vi "InitializeMotorsXYZR_V2.vi"(0 "COM PORT Array IN":refnum<visa-resource-name>[](array[refnum]), 1 "STEP SP Array IN":i32[](array[numeric]), 2 "XYZ in RANGE Array IN":bool[](array[boolean]), 3 "XYZR VEL PV Array IN":i32[](array[numeric]), 4 "RUNHOLDArray IN":i32[](array[numeric]), 5 "Error Array IN":errorcluster[](array[cluster]), 6 "ZR Max Min array":dbl[](array[numeric])) -> (13 "XY Max Min array OUT":dbl[](array[numeric]), 14 "COM PORT Array OUT":refnum<visa-resource-name>[](array[refnum]), 15 "STEP SP Array OUT":i32[](array[numeric]), 16 "XYZ in RANGE Array OUT":bool[](array[boolean]), 17 "XYZR VEL PV Array OUT":i32[](array[numeric]), 18 "XYZR MAX MIN POS":i32[](array[numeric]), 19 "Error Array OUT":errorcluster[](array[cluster]))   [LabVIEW 2010]
panel:
  out "R velocity PV step/sec[3]":i32
  out "Z velocity PV step/sec[2]":i32
  out "Y velocity PV step/sec[1]":i32
  out "X velocity PV step/sec[0]":i32
  out "R in Range[3]":bool
  out "Z in Range[2]":bool
  out "Y in Range[1]":bool
  out "X in Range[0]":bool
  out "R Step SP[3]":i32
  out "Z Step SP[2]":i32
  out "Y Step SP[1]":i32 min=-2304000 max=2304000
  out "X Velocity SP step/sec[4]":i32
  out "Y Velocity SP step/sec[5]":i32
  out "Z Velocity SP step/sec[6]":i32
  out "R Velocity SP step/sec[7]":i32
  out "X Step SP[0]":i32 min=-2304000 max=2304000
  out "Z Run Holding %[7]":i32
  out "R Run Current %[6]":i32
  out "R Run Holding %[5]":i32
  out "Y Run Current %[4]":i32
  out "Y Run Holding %[3]":i32
  out "Z Run Current %[2]":i32
  out "X Run Holding %[1]":i32
  out "X Run Current %[0]":i32
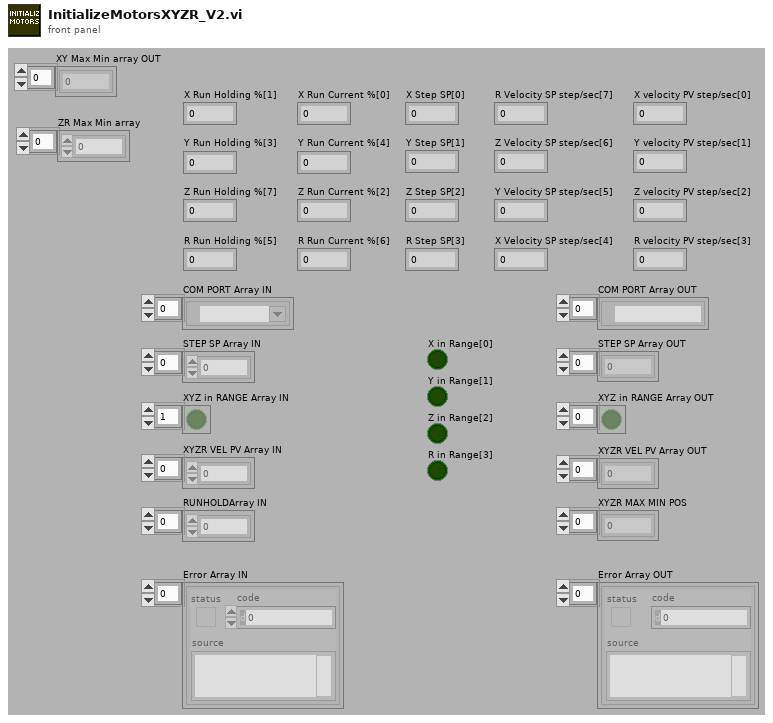
[diagram p1: front panel]
types:
  T1 = cluster{"XYZR VEL PV Array IN[0]":i32, "XYZR VEL PV Array IN[1]":i32, "XYZR VEL PV Array IN[2]":i32, "XYZR VEL PV Array IN[3]":i32, "XYZR VEL PV Array IN[4]":i32, "XYZR VEL PV Array IN[5]":i32, "XYZR VEL PV Array IN[6]":i32, "XYZR VEL PV Array IN[7]":i32, "XYZR VEL PV Array IN[8]":i32}
  T2 = cluster{"RUNHOLDArray IN[0]":i32, "RUNHOLDArray IN[1]":i32, "RUNHOLDArray IN[2]":i32, "RUNHOLDArray IN[3]":i32, "RUNHOLDArray IN[4]":i32, "RUNHOLDArray IN[5]":i32, "RUNHOLDArray IN[6]":i32, "RUNHOLDArray IN[7]":i32, "RUNHOLDArray IN[8]":i32}
  T3 = cluster{"STEP SP Array IN[0]":i32, "STEP SP Array IN[1]":i32, "STEP SP Array IN[2]":i32, "STEP SP Array IN[3]":i32, "STEP SP Array IN[4]":i32, "STEP SP Array IN[5]":i32, "STEP SP Array IN[6]":i32, "STEP SP Array IN[7]":i32, "STEP SP Array IN[8]":i32}
  T4 = cluster{"XYZ in RANGE Array IN[0]":bool, "XYZ in RANGE Array IN[1]":bool, "XYZ in RANGE Array IN[2]":bool, "XYZ in RANGE Array IN[3]":bool, "XYZ in RANGE Array IN[4]":bool, "XYZ in RANGE Array IN[5]":bool, "XYZ in RANGE Array IN[6]":bool, "XYZ in RANGE Array IN[7]":bool, "XYZ in RANGE Array IN[8]":bool}
  T5 = cluster{"RUNHOLDArray IN[0]":i32, "RUNHOLDArray IN[4]":i32}
  T6 = cluster{"RUNHOLDArray IN[2]":i32, "RUNHOLDArray IN[6]":i32}
  T7 = cluster{"RUNHOLDArray IN[1]":i32, "RUNHOLDArray IN[3]":i32}
  T8 = cluster{"RUNHOLDArray IN[7]":i32, "RUNHOLDArray IN[5]":i32}
  T9 = cluster{"STEP SP Array IN[4]":i32, "STEP SP Array IN[5]":i32}
  T10 = cluster{"STEP SP Array IN[6]":i32, "STEP SP Array IN[7]":i32}
  T11 = cluster{"COM PORT Array IN[0]":refnum<visa-resource-name>, "COM PORT Array IN[1]":refnum<visa-resource-name>, "COM PORT Array IN[2]":refnum<visa-resource-name>, "COM PORT Array IN[3]":refnum<visa-resource-name>, "COM PORT Array IN[4]":refnum<visa-resource-name>, "COM PORT Array IN[5]":refnum<visa-resource-name>, "COM PORT Array IN[6]":refnum<visa-resource-name>, "COM PORT Array IN[7]":refnum<visa-resource-name>, "COM PORT Array IN[8]":refnum<visa-resource-name>}
  T12 = cluster{"Error Array IN[0]":errorcluster, "Error Array IN[1]":errorcluster, "Error Array IN[2]":errorcluster, "Error Array IN[3]":errorcluster, "Error Array IN[4]":errorcluster, "Error Array IN[5]":errorcluster, "Error Array IN[6]":errorcluster, "Error Array IN[7]":errorcluster, "Error Array IN[8]":errorcluster}
  T13 = cluster{"ZR Max Min array[0]":dbl, "ZR Max Min array[1]":dbl, "ZR Max Min array[2]":dbl, "ZR Max Min array[3]":dbl, "ZR Max Min array[4]":dbl, "ZR Max Min array[5]":dbl, "ZR Max Min array[6]":dbl, "ZR Max Min array[7]":dbl, "ZR Max Min array[8]":dbl}
  T14 = cluster{"ZR Max Min array[0]":dbl, "ZR Max Min array[2]":dbl}
  T15 = cluster{"ZR Max Min array[1]":dbl, "ZR Max Min array[3]":dbl}
  T16 = cluster{"COM PORT Array IN[0]":refnum<visa-resource-name>, "COM PORT Array IN[2]":refnum<visa-resource-name>}
  T17 = cluster{"Error Array IN[0]":errorcluster, "Error Array IN[2]":errorcluster}
  T18 = cluster{"COM PORT Array IN[1]":refnum<visa-resource-name>, "COM PORT Array IN[3]":refnum<visa-resource-name>}
  T19 = cluster{"Error Array IN[1]":errorcluster, "Error Array IN[3]":errorcluster}
  T20 = enum16{"Stop", "Reset", "Run Current", "Holding Current", "Accel Rate", "Decel Rate", "Move to Relative Position", "Move to Absolute Position", "Echo Mode", "Print Parameter", "Send String", "Microstep Resolution", "Set Current Position", "Max Velocity"}
  T21 = cluster{"[0]":i32, "[1]":i32, "[2]":i32, "[3]":i32, "[4]":i32, "[5]":i32, "[6]":i32, "[7]":i32, "[8]":i32}
  T22 = cluster{"[0]":refnum<visa-resource-name>, "[1]":refnum<visa-resource-name>, "[2]":refnum<visa-resource-name>, "[3]":refnum<visa-resource-name>, "[4]":refnum<visa-resource-name>, "[5]":refnum<visa-resource-name>, "[6]":refnum<visa-resource-name>, "[7]":refnum<visa-resource-name>, "[8]":refnum<visa-resource-name>}
  T23 = cluster{"[0]":errorcluster, "[1]":errorcluster, "[2]":errorcluster, "[3]":errorcluster, "[4]":errorcluster, "[5]":errorcluster, "[6]":errorcluster, "[7]":errorcluster, "[8]":errorcluster}
  T24 = cluster{"[0]":dbl, "[1]":dbl, "[2]":dbl, "[3]":dbl, "[4]":dbl, "[5]":dbl, "[6]":dbl, "[7]":dbl, "[8]":dbl}
  T25 = cluster{"[0]":bool, "[1]":bool, "[2]":bool, "[3]":bool, "[4]":bool, "[5]":bool, "[6]":bool, "[7]":bool, "[8]":bool}
  T26 = cluster{"[0]":dbl, "[0]":dbl, "[1]":dbl, "[1]":dbl}
  T27 = cluster{"[0]":bool, "[1]":bool, "[0]":bool, "[1]":bool}
  T28 = cluster{"[0]":i32, "[0]":i32, "[1]":i32, "[1]":i32, "[0]":i32, "[0]":i32, "[1]":i32, "[1]":i32}
  T29 = cluster{"[0]":i32, "[1]":i32, "[0]":i32, "[1]":i32}
  T30 = cluster{"[0]":refnum<visa-resource-name>, "[0]":refnum<visa-resource-name>, "[1]":refnum<visa-resource-name>, "[1]":refnum<visa-resource-name>}
  T31 = cluster{"[0]":errorcluster, "[0]":errorcluster, "[1]":errorcluster, "[1]":errorcluster}
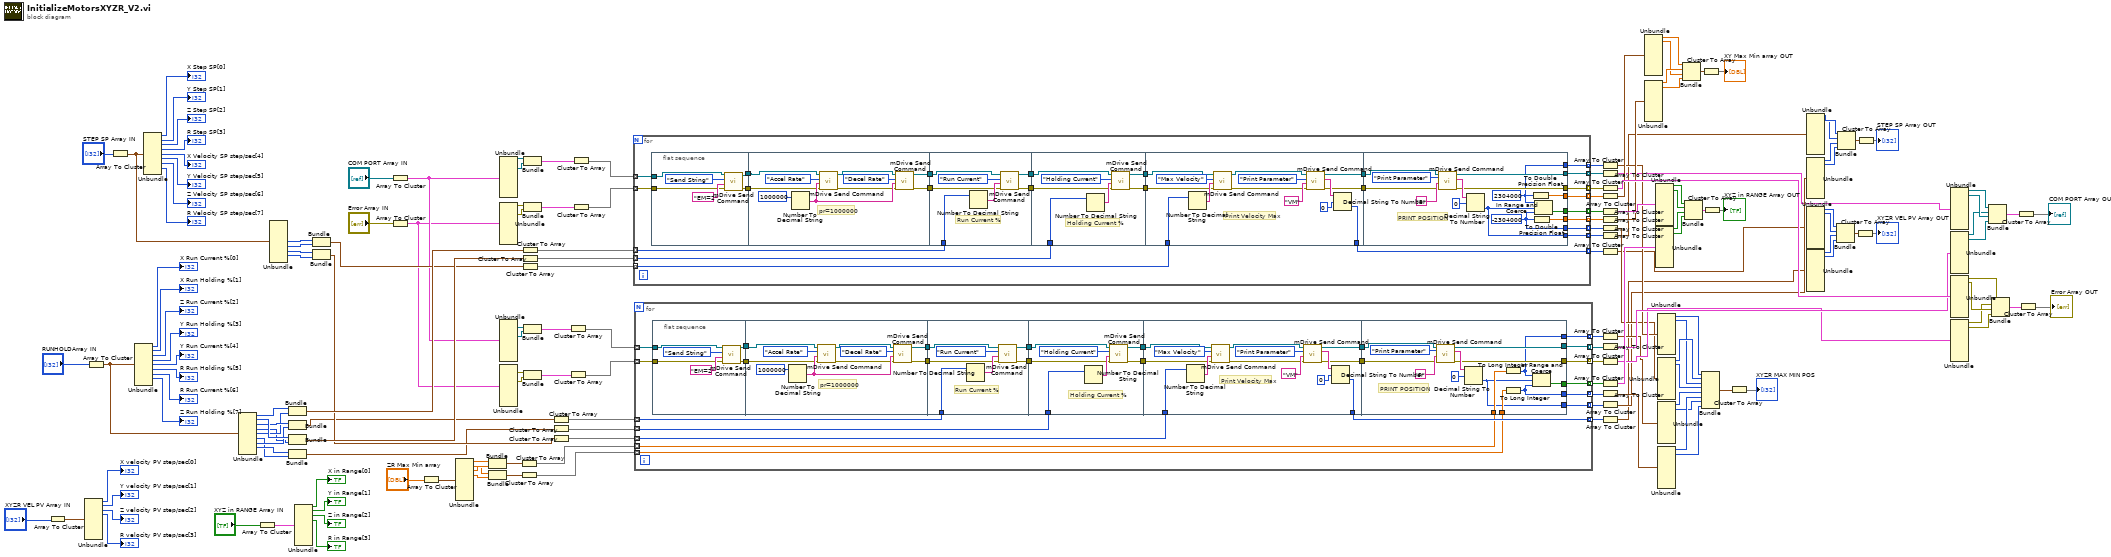
[diagram p0: block diagram]
diagram:
  n1 = Array To Cluster(array="XYZR VEL PV Array IN") -> (cluster=w148:T1)
  n2 = Unbundle(w148) -> ("XYZR VEL PV Array IN[0]"=→"X velocity PV step/sec[0]":i32, "XYZR VEL PV Array IN[1]"=→"Y velocity PV step/sec[1]":i32, "XYZR VEL PV Array IN[2]"=→"Z velocity PV step/sec[2]":i32, "XYZR VEL PV Array IN[3]"=→"R velocity PV step/sec[3]":i32)  [unwired: 5 out]
  n3 = Array To Cluster(array="RUNHOLDArray IN") -> (cluster=w120:T2)
  n4 = Array To Cluster(array="STEP SP Array IN") -> (cluster=w115:T3)
  n5 = Unbundle(w120) -> ("RUNHOLDArray IN[0]"=→"X Run Current %[0]":i32, "RUNHOLDArray IN[1]"=→"X Run Holding %[1]":i32, "RUNHOLDArray IN[2]"=→"Z Run Current %[2]":i32, "RUNHOLDArray IN[3]"=→"Y Run Holding %[3]":i32, "RUNHOLDArray IN[4]"=→"Y Run Current %[4]":i32, "RUNHOLDArray IN[5]"=→"R Run Holding %[5]":i32, "RUNHOLDArray IN[6]"=→"R Run Current %[6]":i32, "RUNHOLDArray IN[7]"=→"Z Run Holding %[7]":i32)  [unwired: 1 out]
  n6 = Unbundle(w115) -> ("STEP SP Array IN[0]"=→"X Step SP[0]":i32, "STEP SP Array IN[1]"=→"Y Step SP[1]":i32, "STEP SP Array IN[2]"=→"Z Step SP[2]":i32, "STEP SP Array IN[3]"=→"R Step SP[3]":i32, "STEP SP Array IN[4]"=→"X Velocity SP step/sec[4]":i32, "STEP SP Array IN[5]"=→"Y Velocity SP step/sec[5]":i32, "STEP SP Array IN[6]"=→"Z Velocity SP step/sec[6]":i32, "STEP SP Array IN[7]"=→"R Velocity SP step/sec[7]":i32)  [unwired: 1 out]
  n7 = Unbundle(w120) -> ("RUNHOLDArray IN[0]"=w113:i32, "RUNHOLDArray IN[1]"=w112:i32, "RUNHOLDArray IN[2]"=w92:i32, "RUNHOLDArray IN[3]"=w89:i32, "RUNHOLDArray IN[4]"=w91:i32, "RUNHOLDArray IN[5]"=w87:i32, "RUNHOLDArray IN[6]"=w90:i32, "RUNHOLDArray IN[7]"=w88:i32)  [unwired: 1 out]
  n8 = Array To Cluster(array="XYZ in RANGE Array IN") -> (cluster=w149:T4)
  n9 = Unbundle(w115) -> ("STEP SP Array IN[4]"=w114:i32, "STEP SP Array IN[5]"=w96:i32, "STEP SP Array IN[6]"=w95:i32, "STEP SP Array IN[7]"=w94:i32)  [unwired: 5 out]
  n10 = Bundle("RUNHOLDArray IN[0]"=w113, "RUNHOLDArray IN[4]"=w91) -> (w119:T5)  [unwired: 1 in]
  n11 = Bundle("RUNHOLDArray IN[2]"=w92, "RUNHOLDArray IN[6]"=w90) -> (w85:T6)  [unwired: 1 in]
  n12 = Bundle("RUNHOLDArray IN[1]"=w112, "RUNHOLDArray IN[3]"=w89) -> (w118:T7)  [unwired: 1 in]
  n13 = Bundle("RUNHOLDArray IN[7]"=w88, "RUNHOLDArray IN[5]"=w87) -> (w84:T8)  [unwired: 1 in]
  n14 = Unbundle(w149) -> ("XYZ in RANGE Array IN[0]"=→"X in Range[0]":bool, "XYZ in RANGE Array IN[1]"=→"Y in Range[1]":bool, "XYZ in RANGE Array IN[2]"=→"Z in Range[2]":bool, "XYZ in RANGE Array IN[3]"=→"R in Range[3]":bool)  [unwired: 5 out]
  n15 = Bundle("STEP SP Array IN[4]"=w114, "STEP SP Array IN[5]"=w96) -> (w111:T9)  [unwired: 1 in]
  n16 = Bundle("STEP SP Array IN[6]"=w95, "STEP SP Array IN[7]"=w94) -> (w93:T10)  [unwired: 1 in]
  n17 = Array To Cluster(array="COM PORT Array IN") -> (cluster=w109:T11)
  n18 = Array To Cluster(array="Error Array IN") -> (cluster=w108:T12)
  n19 = Array To Cluster(array="ZR Max Min array") -> (cluster=w75:T13)
  n20 = Unbundle(w75) -> ("ZR Max Min array[0]"=w74:dbl, "ZR Max Min array[1]"=w72:dbl, "ZR Max Min array[2]"=w73:dbl, "ZR Max Min array[3]"=w71:dbl)  [unwired: 5 out]
  n21 = Bundle("ZR Max Min array[0]"=w74, "ZR Max Min array[2]"=w73) -> (w70:T14)  [unwired: 1 in]
  n22 = Bundle("ZR Max Min array[1]"=w72, "ZR Max Min array[3]"=w71) -> (w69:T15)  [unwired: 1 in]
  n23 = Unbundle(w109) -> ("COM PORT Array IN[0]"=w107:refnum<visa-resource-name>, "COM PORT Array IN[2]"=w80:refnum<visa-resource-name>)  [unwired: 7 out]
  n24 = Unbundle(w108) -> ("Error Array IN[0]"=w106:errorcluster, "Error Array IN[2]"=w79:errorcluster)  [unwired: 7 out]
  n25 = Unbundle(w109) -> ("COM PORT Array IN[1]"=w78:refnum<visa-resource-name>, "COM PORT Array IN[3]"=w105:refnum<visa-resource-name>)  [unwired: 7 out]
  n26 = Unbundle(w108) -> ("Error Array IN[1]"=w77:errorcluster, "Error Array IN[3]"=w81:errorcluster)  [unwired: 7 out]
  n27 = Cluster To Array(cluster=w70) -> (array=w68:dbl[])
  n28 = Cluster To Array(cluster=w69) -> (array=w67:dbl[])
  n29 = Cluster To Array(cluster=w119) -> (array=w117:i32[])
  n30 = Cluster To Array(cluster=w118) -> (array=w116:i32[])
  n31 = Cluster To Array(cluster=w111) -> (array=w110:i32[])
  n32 = Bundle("COM PORT Array IN[0]"=w107, "COM PORT Array IN[2]"=w80) -> (w104:T16)  [unwired: 1 in]
  n33 = Bundle("Error Array IN[0]"=w106, "Error Array IN[2]"=w79) -> (w102:T17)  [unwired: 1 in]
  n34 = Bundle("COM PORT Array IN[1]"=w78, "COM PORT Array IN[3]"=w105) -> (w100:T18)  [unwired: 1 in]
  n35 = Bundle("Error Array IN[1]"=w77, "Error Array IN[3]"=w81) -> (w99:T19)  [unwired: 1 in]
  n36 = Cluster To Array(cluster=w85) -> (array=w82:i32[])
  n37 = Cluster To Array(cluster=w84) -> (array=w83:i32[])
  n38 = Cluster To Array(cluster=w93) -> (array=w86:i32[])
  n39 = Cluster To Array(cluster=w100) -> (array=w97:refnum<visa-resource-name>[])
  n40 = Cluster To Array(cluster=w99) -> (array=w98:errorcluster[])
  n41 = Cluster To Array(cluster=w104) -> (array=w103:refnum<visa-resource-name>[])
  n42 = Cluster To Array(cluster=w102) -> (array=w101:errorcluster[])
  n43 = for {
    tunnel: w103 -> [w186] mode=indexing
    tunnel: w101 -> [w185] mode=indexing
    tunnel: w117 -> [w182] mode=indexing
    tunnel: w116 -> [w179] mode=indexing
    tunnel: w110 -> [w176] mode=indexing
    tunnel: [w173] -> w65 mode=indexing
    tunnel: [w172] -> w63 mode=indexing
    tunnel: [w171] -> w62 mode=indexing
    tunnel: [w170] -> w66 mode=indexing
    tunnel: [w169] -> w61 mode=indexing
    tunnel: [w168] -> w60 mode=indexing
    tunnel: [w167] -> w59 mode=indexing
    tunnel: [w166] -> w58 mode=indexing
    tunnel: [w165] -> w64 mode=indexing
    n44 = flat-sequence {
      tunnel: [w192] -> w188
      tunnel: [w191] -> w187
      tunnel: w186 -> [w190]
      tunnel: w185 -> [w189]
      tunnel: w188 -> [w197]
      tunnel: w187 -> [w198]
      tunnel: [w196] -> w184
      tunnel: [w195] -> w183
      tunnel: w184 -> [w208]
      tunnel: w183 -> [w209]
      tunnel: w182 -> [w207]
      tunnel: [w206] -> w181
      tunnel: [w205] -> w180
      tunnel: w181 -> [w216]
      tunnel: w180 -> [w215]
      tunnel: w179 -> [w214]
      tunnel: [w213] -> w178
      tunnel: [w212] -> w177
      tunnel: w178 -> [w223]
      tunnel: w177 -> [w224]
      tunnel: w176 -> [w222]
      tunnel: [w221] -> w175
      tunnel: [w220] -> w174
      tunnel: [w219] -> w173
      tunnel: w175 -> [w242]
      tunnel: w174 -> [w241]
      tunnel: [w240] -> w168
      tunnel: [w239] -> w167
      tunnel: [w238] -> w171
      tunnel: [w237] -> w172
      tunnel: [w236] -> w166
      tunnel: [w235] -> w170
      tunnel: [w234] -> w169
      tunnel: [w233] -> w165
      frame #0 {
        n45 = call "mDrive Send Command.vi"("error in (no error)"=w189, "Extra"="EM=2", "Command"=T20."Send String", "VISA resource name"=w190) -> ("error out"=w192:errorcluster, "VISA resource name out"=w191:refnum<visa-resource-name>)  [unwired: 3 in, 1 out]
      }
      frame #1 {
        # "pr=1000000"
        n46 = Number To Decimal String(number=1000000) -> (decimal integer string=w200:string)  [unwired: 1 in]
        n47 = call "mDrive Send Command.vi"("error in (no error)"=w197, "Extra"=w200, "Command"=T20."Accel Rate", "VISA resource name"=w198) -> ("error out"=w199:errorcluster, "VISA resource name out"=w204:refnum<visa-resource-name>)  [unwired: 3 in, 1 out]
        n48 = call "mDrive Send Command.vi"("error in (no error)"=w199, "Extra"=w200, "Command"=T20."Decel Rate", "VISA resource name"=w204) -> ("error out"=w195:errorcluster, "VISA resource name out"=w196:refnum<visa-resource-name>)  [unwired: 3 in, 1 out]
      }
      frame #2 {
        # "Run Current %"
        n49 = Number To Decimal String(number=w207) -> (decimal integer string=w210:string)  [unwired: 1 in]
        n50 = call "mDrive Send Command.vi"("error in (no error)"=w209, "Extra"=w210, "Command"=T20."Run Current", "VISA resource name"=w208) -> ("error out"=w206:errorcluster, "VISA resource name out"=w205:refnum<visa-resource-name>)  [unwired: 3 in, 1 out]
      }
      frame #3 {
        # "Holding Current %"
        n51 = Number To Decimal String(number=w214) -> (decimal integer string=w217:string)  [unwired: 1 in]
        n52 = call "mDrive Send Command.vi"("error in (no error)"=w216, "Extra"=w217, "Command"=T20."Holding Current", "VISA resource name"=w215) -> ("error out"=w212:errorcluster, "VISA resource name out"=w213:refnum<visa-resource-name>)  [unwired: 3 in, 1 out]
      }
      frame #4 {
        # "Print Velocity Max"
        n53 = Number To Decimal String(number=w222) -> (decimal integer string=w228:string)  [unwired: 1 in]
        n54 = call "mDrive Send Command.vi"("error in (no error)"=w224, "Extra"=w228, "Command"=T20."Max Velocity", "VISA resource name"=w223) -> ("error out"=w229:errorcluster, "VISA resource name out"=w225:refnum<visa-resource-name>)  [unwired: 3 in, 1 out]
        n55 = call "mDrive Send Command.vi"("error in (no error)"=w229, "Extra"="VM", "Command"=T20."Print Parameter", "VISA resource name"=w225) -> ("error out"=w220:errorcluster, "read buffer"=w227:string, "VISA resource name out"=w221:refnum<visa-resource-name>)  [unwired: 3 in]
        n56 = Decimal String To Number(string=w227, offset=0) -> (number=w219:i32)  [unwired: 1 in, 1 out]
      }
      frame #5 {
        w237 = -2304000 ("lower limit")
        w236 = 2304000 ("upper limit")
        # "PRINT POSITION"
        n57 = call "mDrive Send Command.vi"("error in (no error)"=w241, "Extra"="P", "Command"=T20."Print Parameter", "VISA resource name"=w242) -> ("error out"=w240:errorcluster, "read buffer"=w243:string, "VISA resource name out"=w239:refnum<visa-resource-name>)  [unwired: 3 in]
        n58 = Decimal String To Number(string=w243, offset=0) -> (number=w233:i32)  [unwired: 1 in, 1 out]
        n59 = To Double Precision Float(number=w236) -> (double precision float=w234:dbl)
        n60 = To Double Precision Float(number=w237) -> (double precision float=w238:dbl)
        n61 = In Range and Coerce(upper limit=w236, x=w233, lower limit=w237) -> (In Range?=w235:bool)  [unwired: 1 out]
      }
    }
  }
  n62 = for {
    tunnel: [w260] -> w51 mode=indexing
    tunnel: w98 -> [w259] mode=indexing
    tunnel: w97 -> [w258] mode=indexing
    tunnel: w86 -> [w255] mode=indexing
    tunnel: w82 -> [w257] mode=indexing
    tunnel: w83 -> [w256] mode=indexing
    tunnel: [w254] -> w48 mode=indexing
    tunnel: w68 -> [w253] mode=indexing
    tunnel: w67 -> [w252] mode=indexing
    tunnel: [w251] -> w54 mode=indexing
    tunnel: [w250] -> w53 mode=indexing
    tunnel: [w249] -> w52 mode=indexing
    tunnel: [w248] -> w50 mode=indexing
    tunnel: [w247] -> w49 mode=indexing
    n63 = flat-sequence {
      tunnel: [w274] -> w270
      tunnel: [w273] -> w269
      tunnel: w259 -> [w272]
      tunnel: w258 -> [w271]
      tunnel: w270 -> [w279]
      tunnel: w269 -> [w280]
      tunnel: [w278] -> w268
      tunnel: [w277] -> w267
      tunnel: w268 -> [w290]
      tunnel: w267 -> [w291]
      tunnel: [w289] -> w266
      tunnel: [w288] -> w265
      tunnel: w257 -> [w287]
      tunnel: w266 -> [w298]
      tunnel: w265 -> [w297]
      tunnel: [w296] -> w264
      tunnel: [w295] -> w263
      tunnel: w256 -> [w294]
      tunnel: w264 -> [w305]
      tunnel: w263 -> [w306]
      tunnel: [w304] -> w254
      tunnel: [w303] -> w262
      tunnel: [w302] -> w261
      tunnel: w255 -> [w301]
      tunnel: w262 -> [w324]
      tunnel: w261 -> [w323]
      tunnel: [w322] -> w249
      tunnel: [w321] -> w250
      tunnel: [w320] -> w260
      tunnel: [w319] -> w251
      tunnel: [w318] -> w248
      tunnel: w253 -> [w317]
      tunnel: w252 -> [w316]
      tunnel: [w315] -> w247
      frame #0 {
        n64 = call "mDrive Send Command.vi"("error in (no error)"=w272, "Extra"="EM=2", "Command"=T20."Send String", "VISA resource name"=w271) -> ("error out"=w274:errorcluster, "VISA resource name out"=w273:refnum<visa-resource-name>)  [unwired: 3 in, 1 out]
      }
      frame #1 {
        # "pr=1000000"
        n65 = Number To Decimal String(number=1000000) -> (decimal integer string=w282:string)  [unwired: 1 in]
        n66 = call "mDrive Send Command.vi"("error in (no error)"=w279, "Extra"=w282, "Command"=T20."Accel Rate", "VISA resource name"=w280) -> ("error out"=w281:errorcluster, "VISA resource name out"=w286:refnum<visa-resource-name>)  [unwired: 3 in, 1 out]
        n67 = call "mDrive Send Command.vi"("error in (no error)"=w281, "Extra"=w282, "Command"=T20."Decel Rate", "VISA resource name"=w286) -> ("error out"=w277:errorcluster, "VISA resource name out"=w278:refnum<visa-resource-name>)  [unwired: 3 in, 1 out]
      }
      frame #2 {
        # "Run Current %"
        n68 = Number To Decimal String(number=w287) -> (decimal integer string=w292:string)  [unwired: 1 in]
        n69 = call "mDrive Send Command.vi"("error in (no error)"=w291, "Extra"=w292, "Command"=T20."Run Current", "VISA resource name"=w290) -> ("error out"=w289:errorcluster, "VISA resource name out"=w288:refnum<visa-resource-name>)  [unwired: 3 in, 1 out]
      }
      frame #3 {
        # "Holding Current %"
        n70 = Number To Decimal String(number=w294) -> (decimal integer string=w299:string)  [unwired: 1 in]
        n71 = call "mDrive Send Command.vi"("error in (no error)"=w298, "Extra"=w299, "Command"=T20."Holding Current", "VISA resource name"=w297) -> ("error out"=w295:errorcluster, "VISA resource name out"=w296:refnum<visa-resource-name>)  [unwired: 3 in, 1 out]
      }
      frame #4 {
        # "Print Velocity Max"
        n72 = Number To Decimal String(number=w301) -> (decimal integer string=w310:string)  [unwired: 1 in]
        n73 = call "mDrive Send Command.vi"("error in (no error)"=w306, "Extra"=w310, "Command"=T20."Max Velocity", "VISA resource name"=w305) -> ("error out"=w311:errorcluster, "VISA resource name out"=w307:refnum<visa-resource-name>)  [unwired: 3 in, 1 out]
        n74 = call "mDrive Send Command.vi"("error in (no error)"=w311, "Extra"="VM", "Command"=T20."Print Parameter", "VISA resource name"=w307) -> ("error out"=w302:errorcluster, "read buffer"=w309:string, "VISA resource name out"=w303:refnum<visa-resource-name>)  [unwired: 3 in]
        n75 = Decimal String To Number(string=w309, offset=0) -> (number=w304:i32)  [unwired: 1 in, 1 out]
      }
      frame #5 {
        # "PRINT POSITION"
        n76 = call "mDrive Send Command.vi"("error in (no error)"=w323, "Extra"="P", "Command"=T20."Print Parameter", "VISA resource name"=w324) -> ("error out"=w322:errorcluster, "read buffer"=w325:string, "VISA resource name out"=w321:refnum<visa-resource-name>)  [unwired: 3 in]
        n77 = Decimal String To Number(string=w325, offset=0) -> (number=w315:i32)  [unwired: 1 in, 1 out]
        n78 = To Long Integer(number=w317) -> (32bit integer=w319:i32)
        n79 = To Long Integer(number=w316) -> (32bit integer=w318:i32)
        n80 = In Range and Coerce(upper limit=w319, x=w315, lower limit=w318) -> (In Range?=w320:bool)  [unwired: 1 out]
      }
    }
  }
  n81 = Array To Cluster(array=w58) -> (cluster=w33:T21)
  n82 = Array To Cluster(array=w59) -> (cluster=w1:T22)
  n83 = Array To Cluster(array=w60) -> (cluster=w44:T23)
  n84 = Array To Cluster(array=w61) -> (cluster=w40:T24)
  n85 = Array To Cluster(array=w66) -> (cluster=w57:T25)
  n86 = Array To Cluster(array=w62) -> (cluster=w39:T24)
  n87 = Array To Cluster(array=w63) -> (cluster=w32:T21)
  n88 = Array To Cluster(array=w64) -> (cluster=w21:T21)
  n89 = Array To Cluster(array=w65) -> (cluster=w18:T21)
  n90 = Array To Cluster(array=w54) -> (cluster=w31:T21)
  n91 = Array To Cluster(array=w53) -> (cluster=w43:T22)
  n92 = Array To Cluster(array=w52) -> (cluster=w42:T23)
  n93 = Array To Cluster(array=w51) -> (cluster=w47:T25)
  n94 = Array To Cluster(array=w50) -> (cluster=w30:T21)
  n95 = Array To Cluster(array=w49) -> (cluster=w20:T21)
  n96 = Array To Cluster(array=w48) -> (cluster=w19:T21)
  n97 = Unbundle(w40) -> ("[0]"=w38:dbl, "[1]"=w35:dbl)  [unwired: 7 out]
  n98 = Unbundle(w39) -> ("[0]"=w37:dbl, "[1]"=w36:dbl)  [unwired: 7 out]
  n99 = Unbundle(w57) -> ("[0]"=w56:bool, "[1]"=w55:bool)  [unwired: 7 out]
  n100 = Unbundle(w47) -> ("[0]"=w45:bool, "[1]"=w46:bool)  [unwired: 7 out]
  n101 = Unbundle(w33) -> ("[0]"=w29:i32, "[1]"=w27:i32)  [unwired: 7 out]
  n102 = Unbundle(w32) -> ("[0]"=w28:i32, "[1]"=w26:i32)  [unwired: 7 out]
  n103 = Unbundle(w31) -> ("[0]"=w25:i32, "[1]"=w22:i32)  [unwired: 7 out]
  n104 = Unbundle(w30) -> ("[0]"=w24:i32, "[1]"=w23:i32)  [unwired: 7 out]
  n105 = Bundle("[0]"=w38, "[0]"=w37, "[1]"=w35, "[1]"=w36) -> (w41:T26)  [unwired: 1 in]
  n106 = Bundle("[0]"=w56, "[1]"=w55, "[0]"=w45, "[1]"=w46) -> (w131:T27)  [unwired: 1 in]
  n107 = Bundle("[0]"=w29, "[0]"=w28, "[1]"=w27, "[1]"=w26, "[0]"=w25, "[0]"=w24, "[1]"=w22, "[1]"=w23) -> (w125:T28)  [unwired: 1 in]
  n108 = Cluster To Array(cluster=w41) -> (array=→"XY Max Min array OUT":dbl[])
  n109 = Cluster To Array(cluster=w131) -> (array=→"XYZ in RANGE Array OUT":bool[])
  n110 = Cluster To Array(cluster=w125) -> (array=→"XYZR MAX MIN POS":i32[])
  n111 = Unbundle(w21) -> ("[0]"=w17:i32, "[1]"=w16:i32)  [unwired: 7 out]
  n112 = Unbundle(w20) -> ("[0]"=w15:i32, "[1]"=w14:i32)  [unwired: 7 out]
  n113 = Unbundle(w18) -> ("[0]"=w13:i32, "[1]"=w12:i32)  [unwired: 7 out]
  n114 = Unbundle(w19) -> ("[0]"=w11:i32, "[1]"=w10:i32)  [unwired: 7 out]
  n115 = Bundle("[0]"=w13, "[1]"=w12, "[0]"=w11, "[1]"=w10) -> (w129:T29)  [unwired: 1 in]
  n116 = Bundle("[0]"=w17, "[1]"=w16, "[0]"=w15, "[1]"=w14) -> (w127:T29)  [unwired: 1 in]
  n117 = Cluster To Array(cluster=w129) -> (array=→"XYZR VEL PV Array OUT":i32[])
  n118 = Cluster To Array(cluster=w127) -> (array=→"STEP SP Array OUT":i32[])
  n119 = Unbundle(w1) -> ("[0]"=w9:refnum<visa-resource-name>, "[1]"=w8:refnum<visa-resource-name>)  [unwired: 7 out]
  n120 = Unbundle(w43) -> ("[0]"=w7:refnum<visa-resource-name>, "[1]"=w6:refnum<visa-resource-name>)  [unwired: 7 out]
  n121 = Unbundle(w44) -> ("[0]"=w5:errorcluster, "[1]"=w4:errorcluster)  [unwired: 7 out]
  n122 = Unbundle(w42) -> ("[0]"=w3:errorcluster, "[1]"=w2:errorcluster)  [unwired: 7 out]
  n123 = Bundle("[0]"=w9, "[0]"=w7, "[1]"=w8, "[1]"=w6) -> (w164:T30)  [unwired: 1 in]
  n124 = Bundle("[0]"=w5, "[0]"=w3, "[1]"=w4, "[1]"=w2) -> (w162:T31)  [unwired: 1 in]
  n125 = Cluster To Array(cluster=w164) -> (array=→"COM PORT Array OUT":refnum<visa-resource-name>[])
  n126 = Cluster To Array(cluster=w162) -> (array=→"Error Array OUT":errorcluster[])
